vi "Write Active Plot.vi"(8 "error in (no error)":errorcluster, 9 "Active Plot":i32, 11 "3D Quiver.lvclass in":refnum<class "3D Quiver.lvclass">) -> (0 "error out":errorcluster, 3 "3D Quiver.lvclass out":refnum<class "3D Quiver.lvclass">)   [LabVIEW 2017, in "3D Quiver.lvclass"]
uses:
  <vilib>/Math Plots/3D Math Plots/3D Quiver/3D Quiver/3D Quiver.lvclass
  <vilib>/Math Plots/3D Math Plots/3D Quiver/3D Quiver/3D Quiver.lvclass/3D Quiver.ctl
  <vilib>/Math Plots/3D Math Plots/3D Plot/3D Plot/3D Plot.lvclass
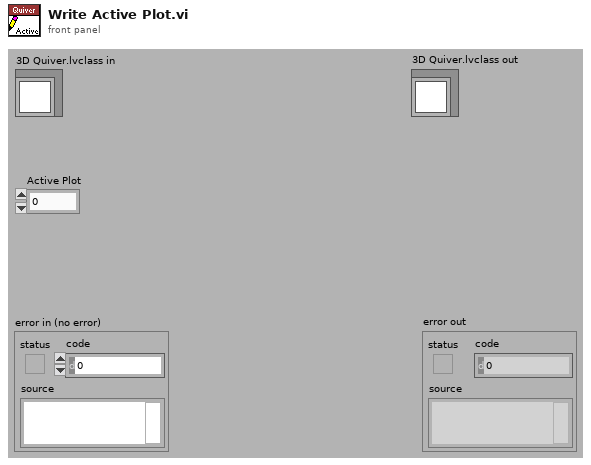
[diagram p1: front panel]
types:
  T1 = typedef "3D Quiver.lvclass/3D Quiver Property Array.ctl" = T2[]
  T2 = typedef "3D Quiver.lvclass/3D Quiver Property.ctl" = cluster{"General Property":cluster{"Plot Name":string, "Coordinate System":enum16{"Cartesian", "Cylindrical", "Spherical"}, "Opacity":sgl}, "Projection Property":cluster{"Draw XY":bool, "Draw YZ":bool, "Draw XZ":bool}, "Plot Property":cluster{"Line Style":T3, "Line Width":sgl, "Line Color":u32, "Antialiasing":bool, "Color Ramp Cluster":T4}, "Quiver Property":cluster{"Quvier Mode":enum16{"Quiver", "Quiver with surface"}, "Quiver Size":sgl, "Quiver Length":sgl}}
  T3 = typedef "3D Plot.lvclass/Line Type.ctl" = enum16{"None", "Solid", "Dash", "Dot", "Dash Dot"}
  T4 = typedef "3D Plot.lvclass/Color Ramp Cluster.ctl" = cluster{"Color Ramp Style":enum16{"None", "Shaded", "Color spectrum", "Grey scale", "Custom"}, "Color Ramp Array":u32[], "Color Ramp Index":i32[], "Interpolate?":bool, "Logarithm?":bool}
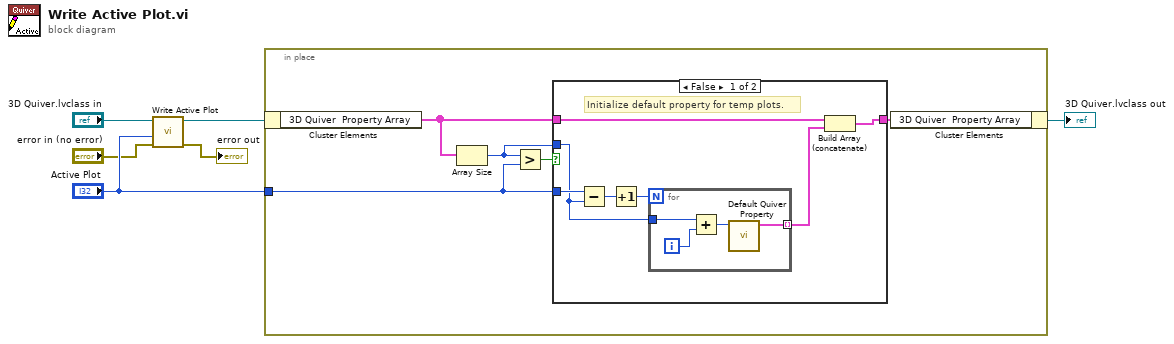
[diagram p0: block diagram]
diagram:
  n1 = call-parent "Write Active Plot.vi"("error in (no error)"="error in (no error)", "Active Plot"="Active Plot", "3D Plot.lvclass in"="3D Quiver.lvclass in") -> ("error out"=→"error out":errorcluster, "3D Plot.lvclass out"=w6:refnum<class "3D Quiver.lvclass">)  [unwired: 7 in]
  n2 = in-place {
    in-place-border: "Active Plot" -> [w8]
    n3 = in-place-cluster #1(w6) -> ("3D Quiver  Property Array"=w10:T1)
    n4 = Array Size(array=w10) -> (size(s)=w7:i32)
    n5 = Greater?(x=w7, y=w8) -> (0:w11:bool)
    n6 = case shown="False" w11 {
      tunnel: [w16 w23] -> w9
      tunnel: w10 -> [w18 w23]
      tunnel: w7 -> [w12 _]
      tunnel: w8 -> [w13 _]
      frame False {
        # "Initialize default property for temp plots."
        n7 = Subtract(x=w13, y=w12) -> (x-y=w15:i32)
        n8 = Increment(x=w15) -> (x+1=w14:i32)
        n9 = for {
          N: w14 -> [_]
          tunnel: w12 -> [w21]
          tunnel: [w19] -> w17 mode=indexing
          i -> [w22]
          n10 = Add(x=w21, y=w22) -> (x+y=w20:i32)
          n11 = call <vilib>:"Default Quiver Property.vi"("Plot ID"=w20) -> ("Default Property"=w19:T2)  [unwired: 10 in]
        }
        n12 = Build Array (concatenate)(w18, w17) -> (w16:T1)
      }
      frame True {
      }
    }
    n13 = in-place-cluster #1("3D Quiver  Property Array"=w9) -> (→"3D Quiver.lvclass out":refnum<class "3D Quiver.lvclass">)
  }
